vi "信号采集.vi"(0 "Boolean":bool) -> (1 "mono 16-bit":i16[](array[numeric]), 2 "波形图":i16[](graph))   [LabVIEW 2013]
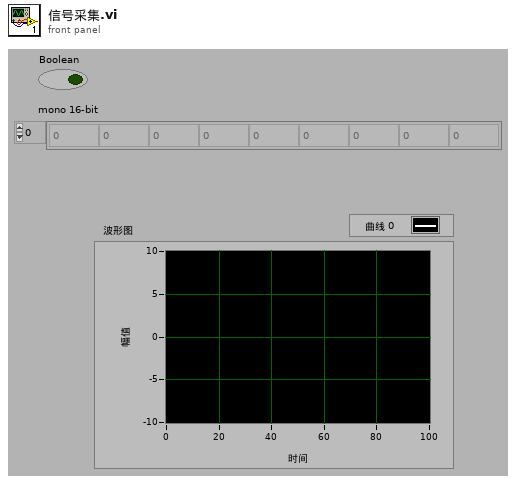
[diagram p1: front panel]
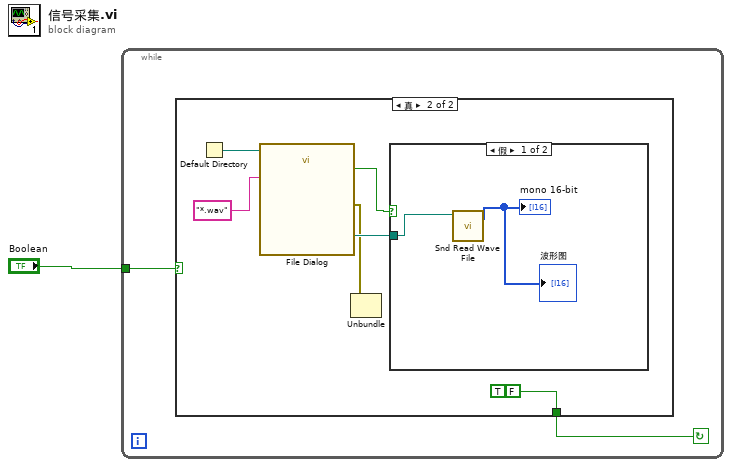
[diagram p0: block diagram]
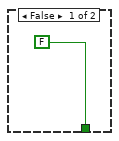
[diagram p2: hidden frame]
diagram:
  n1 = while {
    tunnel: "Boolean" -> [w2]
    stop <- w3 continue-if-true
    n2 = case shown="真" w2 {
      tunnel: [FALSE FALSE] -> w3
      frame False {
      }
      frame True {
        (unwired) TRUE
        n3 = Default Directory() -> (w9:path)
        n4 = call "File Dialog"("start path"=w9, "pattern (all files)"="*.wav") -> ("selected path"=w7:path, "exists"=w5:bool, "error out"=w6:errorcluster)  [unwired: 10 in, 1 out]
        n5 = Unbundle(w6) -> ()  [unwired: 3 out]
        n6 = case shown="假" w5 {
          tunnel: w7 -> [w11 _]
          frame False {
            n7 = call <vilib>:"Snd Read Wave File.vi"("wave file path"=w11) -> ("mono 16-bit"=→"mono 16-bit" →"波形图":i16[])  [unwired: 4 in, 6 out]
          }
          frame True {
          }
        }
      }
    }
  }
